vi "Get Plugin Paths.vi"(8 "error in (no error)":errorcluster, 11 "MeasurementService in":refnum<class "MeasurementPluginService.lvclass">) -> (0 "error out":errorcluster, 2 "Plugin Paths":T1, 3 "MeasurementService out":refnum<class "MeasurementPluginService.lvclass">)   [LabVIEW 2020, in "MeasurementLink Measurement Server.lvlib" / "MeasurementPluginService.lvclass"]
uses:
  MeasurementPluginService.lvclass
  Plugin Paths.ctl
  MeasurementPluginService.lvclass/MeasurementPluginService.ctl
  Helpers/Error Strings Global.vi
  MeasurementLink Measurement Server.lvlib
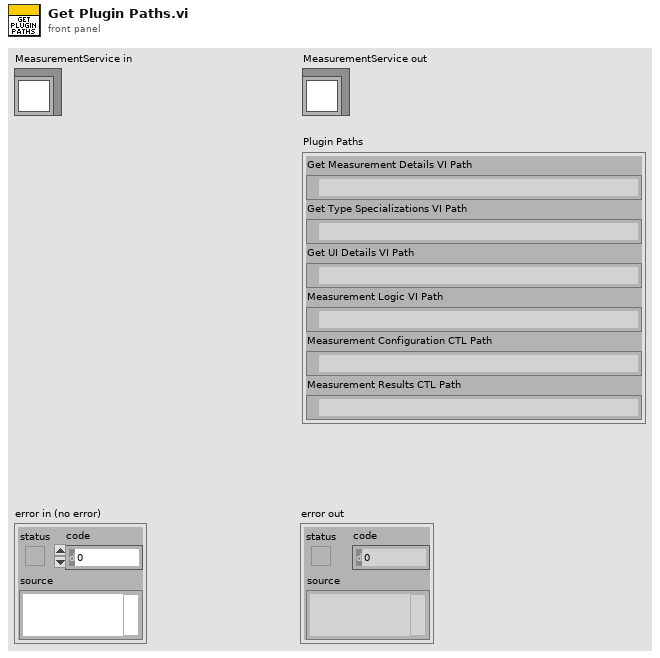
[diagram p1: front panel]
types:
  T1 = typedef "MeasurementLink Measurement Server.lvlib/MeasurementPluginService.lvclass/Plugin Paths.ctl" = cluster{"Get Measurement Details VI Path":path, "Get Type Specializations VI Path":path, "Get UI Details VI Path":path, "Measurement Logic VI Path":path, "Measurement Configuration CTL Path":path, "Measurement Results CTL Path":path}
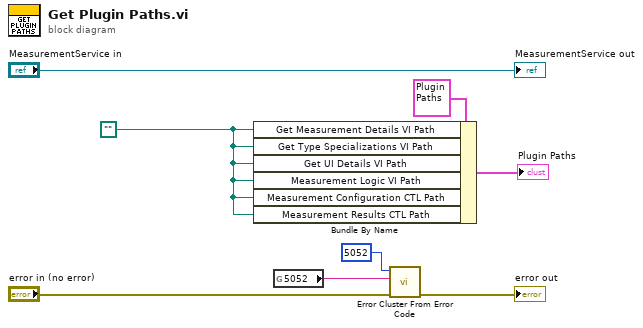
[diagram p0: block diagram]
diagram:
  w2 = path ""
  n1 = Bundle By Name(cluster=T1 {"Get Measurement Details VI Path"=path "", "Get Type Specializations VI Path"=path "", "Get UI Details VI Path"=path "", "Measurement Logic VI Path"=path "", "Measurement Configuration CTL Path"=path "", "Measurement Results CTL Path"=path ""} ("Plugin Paths"), "Get Measurement Details VI Path"=w2, "Get Type Specializations VI Path"=w2, "Get UI Details VI Path"=w2, "Measurement Logic VI Path"=w2, "Measurement Configuration CTL Path"=w2, "Measurement Results CTL Path"=w2) -> (→"Plugin Paths":T1)
  n2 = global read "Error Strings Global.vi" "5052"() -> (w1:string)
  n3 = call <vilib>:"Error Cluster From Error Code.vi"("error in (no error)"="error in (no error)", "error message (\"\")"=w1, "error code (0)"=5052) -> ("error out"=→"error out":errorcluster)  [unwired: 6 in]
  "MeasurementService out" <- "MeasurementService in"
